vi "interpolate-phase.vi"(6 "Ready For Output":bool, 8 "Input Valid":bool, 11 "phase in":fxp<+,26,1>) -> (0 "Output Valid":bool, 2 "rising edge!":bool, 3 "pulse idx out":u8, 4 "Ready For Input":bool=TRUE, 5 "transition":bool)   [LabVIEW 2018, in "SCTL.lvlib"]
doc: "This VI is used in four wire handshake."
uses:
  SCTL.lvlib
  <vilib>/rvi/FXPMathLib/FxpDiv/subVIs/nifxpmath_Div_SimConfig.ctl
  <vilib>/rvi/FXPMathLib/FxpDiv/simVIs/DllFxpDivTemp_sub.vi
  <vilib>/rvi/FXPMathLib/FxpSub/XNode/nifxpmath_Sub.xnode
  <vilib>/rvi/FXPMathLib/FxpMul/XNode/nifxpmath_Multiplier.xnode
  <vilib>/rvi/FXPMathLib/FxpAdd/XNode/nifxpmath_Add.xnode
  <vilib>/rvi/FXPMathLib/FxpDiv/XNode/nifxpmath_Div.xnode
  <vilib>/rvi/FXPMathLib/sim/FxpSim.dll
panel:
  # "Inputs"
  # "Outputs"
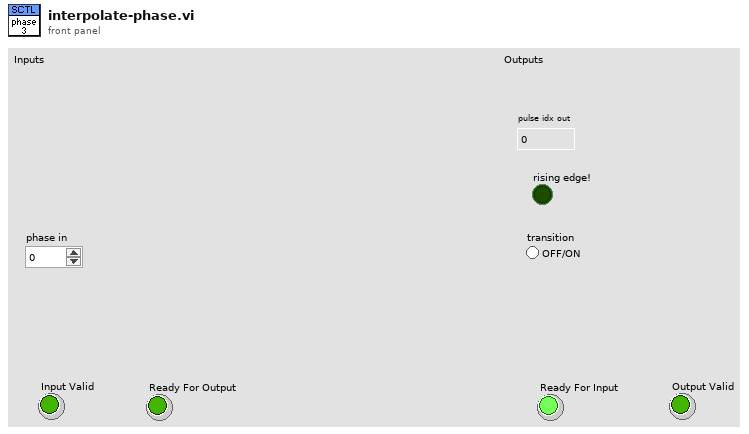
[diagram p1: front panel]
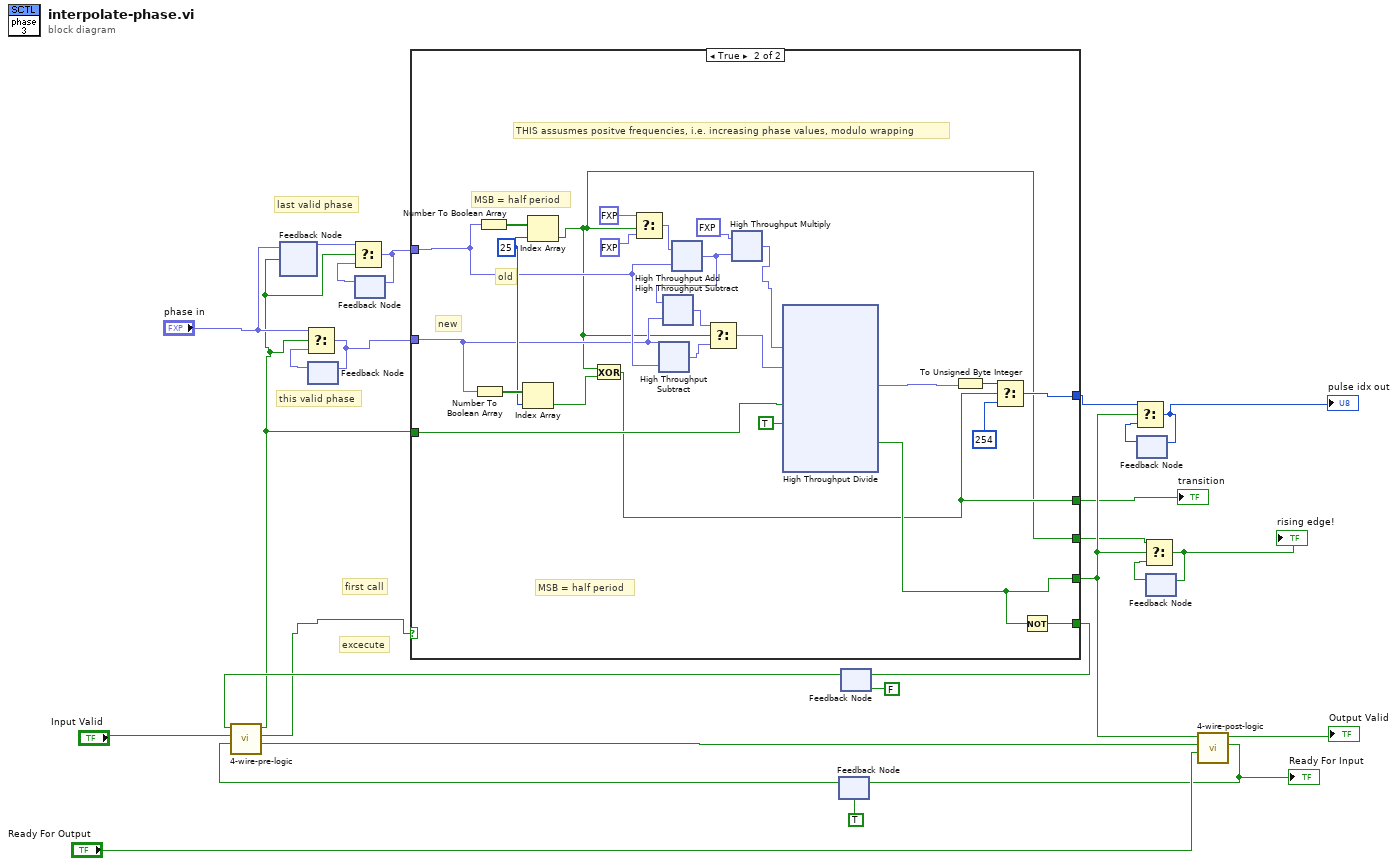
[diagram p0: block diagram]
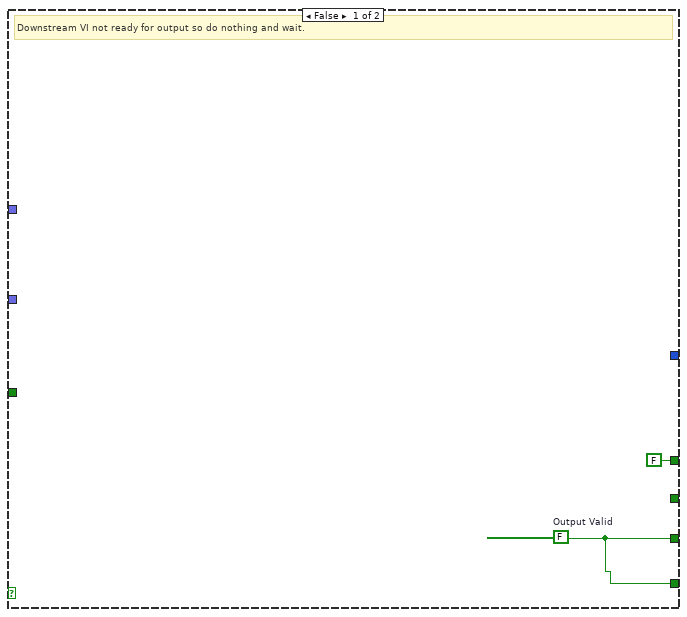
[diagram p2: hidden frame]
diagram:
  # "this valid phase"
  # "last valid phase"
  # "excecute"
  # "first call"
  n1 = feedback #1() -> (w3:fxp<+,26,1>)  [unwired: 1 in]
  n2 = feedback #2() -> (w7:fxp<+,26,1>)  [unwired: 1 in]
  n3 = feedback #3() -> (w1:fxp<+,26,1>)  [unwired: 1 in]
  n4 = feedback #4(TRUE ("x .and. y?")) -> (w23:bool)
  n5 = feedback #5(FALSE ("x .and. y?")) -> (w21:bool)
  n6 = call "4-wire-pre-logic.vi"("ready for input in"=w23, "Input Valid in"="Input Valid", "needs more iter in"=w21) -> ("register state out"=w25:bool, "excecute"=w15:bool, "buffer input!"=w4:bool)  [unwired: 6 in]
  n7 = feedback-in #1("phase in", w4) -> ()
  n8 = Select(t="phase in", s=w4, f=w7) -> (s? t:f=w8:fxp<+,26,1>)
  n9 = feedback-in #2(w8) -> ()
  n10 = Select(t=w3, s=w4, f=w1) -> (s? t:f=w2:fxp<+,26,1>)
  n11 = feedback-in #3(w2) -> ()
  n12 = case shown="True" w15 {
    tunnel: [w28 w41] -> w11
    tunnel: w4 -> [_ w42]
    tunnel: [w28 w43] -> w20
    tunnel: w8 -> [_ w37]
    tunnel: [_ w45] -> w14
    tunnel: [_ w34] -> w10
    tunnel: w2 -> [_ w39]
    tunnel: [FALSE w38] -> w6
    frame False {
      w28 = FALSE  # Output Valid
      # "Downstream VI not ready for output so do nothing and wait."
    }
    frame True {
      w40 = 25 ("index")
      # "THIS assusmes positve frequencies, i.e. increasing phase values, modulo wrapping"
      # "MSB = half period"
      # "MSB = half period"
      # "new"
      # "old"
      n13 = Number To Boolean Array(number=w37) -> (Boolean array=w51:bool[])
      n14 = Number To Boolean Array(number=w39) -> (Boolean array=w50:bool[])
      n15 = Index Array(array=w51, index=w40) -> (element=w46:bool)
      n16 = Index Array(array=w50, index=w40) -> (element=w34:bool)
      n17 = Exclusive Or(1:w46, 2:w34) -> (0:w38:bool)
      n18 = Select(t=fxp<+,1,2> 2.0 ("x"), s=w34, f=fxp<+,1,1> 1.0 ("x")) -> (s? t:f=w47:fxp<+,2,2>)
      n19 = xnode "High Throughput Subtract"("x"=w37, "y"=w39) -> ("x-y"=w35:fxp<+,26,1>)
      n20 = xnode "High Throughput Subtract"("x"=w47, "y"=w39) -> ("x-y"=w31:fxp<+,26,1>)
      n21 = xnode ("High Throughput Add")("x"=w31, "y"=w37) -> ("x+y"=w36:fxp<+,26,1>)
      n22 = Select(t=w36, s=w34, f=w35) -> (s? t:f=w33:fxp<+,26,1>)
      n23 = xnode ("High Throughput Multiply")("x"=fxp<+,8,8> 239.0, "y"=w31) -> ("x*y"=w30:fxp<+,10,8>)
      n24 = xnode "High Throughput Divide"("x"=w30, "y"=w33, "input valid"=w42, "ready for output (T)"=TRUE) -> ("x/y"=w29:fxp<+,8,8>, "output valid"=w41:bool)  [unwired: 1 out]
      n25 = To Unsigned Byte Integer(number=w29) -> (unsigned 8bit integer=w52:u8)
      n26 = Select(t=w52, s=w38, f=u8 254) -> (s? t:f=w45:u8)
      n27 = Not(x=w41) -> (.not. x?=w43:bool)
    }
  }
  "transition" <- w6
  n28 = feedback-in #5(w20) -> ()
  n29 = feedback #6() -> (w24:u8)  [unwired: 1 in]
  n30 = Select(t=w14, s=w11, f=w24) -> (s? t:f=w13:u8)
  "pulse idx out" <- w13
  n31 = feedback-in #6(w13) -> ()
  n32 = feedback #7() -> (w12:bool)  [unwired: 1 in]
  n33 = Select(t=w10, s=w11, f=w12) -> (s? t:f=w9:bool)
  "rising edge!" <- w9
  n34 = feedback-in #7(w9) -> ()
  n35 = call "4-wire-post-logic.vi"("Ready For Output in"="Ready For Output", "register state in"=w25, "output valid in"=w11) -> ("ready for input out"=w17:bool, "output valid out"=→"Output Valid":bool)  [unwired: 7 in]
  "Ready For Input" <- w17
  n36 = feedback-in #4(w17) -> ()
